vi "_Copy IPF Files.vi"   [LabVIEW 2015]
uses:
  Type/_SaveOption.ctl
types:
  T1 = typedef "_SaveOption.ctl" = enum16{"Use Dialog", "Temporary File", "My Tables", "Full Path"}
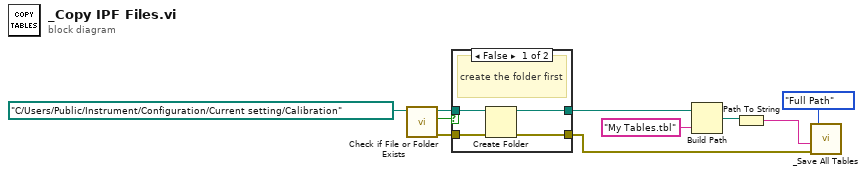
[diagram p0: block diagram]
diagram:
  n1 = call <vilib>:"Check if File or Folder Exists.vi"("path"=path "C:/Users/Public/Instrument/Configuration/Current setting/Calibration" ("base path")) -> ("error out"=w5:errorcluster, "file or folder exists?"=w4:bool, "dup path"=w6:path)  [unwired: 8 in]
  n2 = case shown="False" w4 {
    tunnel: w5 -> [w14 w16]
    tunnel: w6 -> [w13 w15]
    tunnel: [w11 w16] -> w1
    tunnel: [w12 w15] -> w8
    frame False {
      # "create the folder first"
      n3 = Create Folder(path (use dialog)=w13, error in=w14) -> (created path=w12:path, error out=w11:errorcluster)  [unwired: 1 in, 1 out]
    }
    frame True {
      # "Parent folder exists continue on"
    }
  }
  n4 = Build Path(base path=w8, name or relative path="My Tables.tbl") -> (appended path=w2:path)
  n5 = Path To String(path=w2) -> (string=w10:string)
  n6 = call "_Save All Tables.vi"("error in (no error)"=w1, "FilePath(My Table.tbl)"=w10, "SaveOption (Temporary File)"=_SaveOption."Full Path") -> ()  [unwired: 5 out]
